vi "Dashboard Main.vi"() -> ()   [LabVIEW 2015]
uses:
  <vilib>/Utility/miscctls.llb/LVRowAndColumnTypeDef.ctl
  <vilib>/event_ctls.llb/eventvkey.ctl
  <vilib>/Rock Robotics/WPI/Dashboard/WPI_DashboardLogging Global.vi
  <vilib>/Rock Robotics/Network Tables/NT Read Numeric Array.vi
  <vilib>/Rock Robotics/Network Tables/NT Read Boolean.vi
  <vilib>/Utility/config.llb/Write Key (String).vi
  <vilib>/Utility/config.llb/Write Key (I32).vi
  <vilib>/Utility/config.llb/NI_LVConfig.lvlib
panel:
  in  "TCP":refnum<k5>
  in  "Rec Mode":enum32{"Stop", "Record", "Playback"}(radio)
  in  "Vision":u16(ring) items=["Camera Off", "USB Camera SW", "USB Camera HW", "IP Camera"]
  out "Camera IP":string
  out "Image Message":string="Timeout in Camera Communications"
  in  "Dashboard Tab":T1(tab)
  out "TANK":bool
  out "NT Connected":bool
  in  "Camera Settings":T2={"Frame Rate"=30, "Compression"=30, "Size"=1} {"Frame Rate" scale=1.0..30.0; "Size" items=["640x480", "320x240", "160x120"]}
  out "MotorChart R":cluster{"Numeric":dbl, "Numeric":dbl}(graph)
  out "MotorChart L":T3(graph)
  out "MotorSliders R":cluster{"MotorSlide1":dbl, "MotorSlide2":dbl} {"MotorSlide2" scale=-1.0..1.0 scale format="%#_2e"; "MotorSlide1" scale=-1.0..1.0 scale format="%#_2e"}
  out "MotorSliders L":T4 {"MotorSlide4 2" scale=0.0..14.0 scale format="%#_2e"; "MotorSlide2" scale=-1.0..1.0 scale format="%#_2e"; "MotorSlide1" scale=-1.0..1.0 scale format="%#_2e"}
  out "Gyro":dbl(knob) scale=0.0..360.0
  out "JS1 Z":dbl(slide) scale=-1.0..1.0 scale format="%#_2e"
  out "JS1 Graph":cluster{"X":dbl, "Y":dbl}[](graph)
  out "JS1 Buttons":T5
  out "JS2 Z":dbl(slide) scale=-1.0..1.0 scale format="%#_2e"
  out "JS2 Graph":cluster{"X":dbl, "Y":dbl}[](graph)
  out "JS2 Buttons":T5
  out "Mode":T6(ring)=enum."Auto Disabled"
  in  "DB Camera Config":bool
  out "fps":dbl format="%#.1g"
  out "Mbps":dbl format="%#.1g"
  out "Mbps 2":bool
  in  "DB/String 9":string
  in  "DB/String 8":string
  in  "DB/String 7":string
  in  "DB/String 6":string
  in  "DB/String 5":string
  in  "DB/String 4":string
  in  "DB/String 3":string
  in  "DB/String 2":string
  in  "DB/String 1":string
  in  "DB/String 0":string
  in  "DB/Slider 0":dbl(slide) scale=0.0..5.0
  in  "DB/Slider 1":dbl(slide) scale=0.0..5.0
  in  "DB/Slider 2":dbl(slide) scale=0.0..5.0
  in  "DB/Slider 3":dbl(slide) scale=0.0..5.0
  out "DB/LED 3":bool
  out "DB/LED 2":bool
  out "DB/LED 1":bool
  out "DB/LED 0":bool
  in  "DB/Button 3":bool
  in  "DB/Button 2":bool
  in  "DB/Button 1":bool
  in  "DB/Button 0":bool caption="New Name"
  in  "Test Slider":dbl(slide) scale=0.0..100.0 scale format="%#_3g"
  in  "On/Off":bool caption="Solenoid"
  in  "Test Name":u16(ring) items=["Select the test to run..."]
  in  "Test Tree":string(tree)
  in  "Motor":cluster{"Value":dbl, "Enable":bool} {"Value" scale=-1.0..1.0 scale format="%#_3g"}
  out "Progress":T7 {"Test Progress" scale=0.0..100.0}
  in  "Rev/Fwd":cluster{"Forward":bool, "Reverse":bool}
  in  "Test Ring":u16(ring) items=["Monochrome", "Color"]
  out "Cmd Status":string
  in  "Execute Command":bool
  in  "Command Params":string[][](table)
  in  "Command Selection":i32(listbox)
  in  "CheckList":i32(listbox)
  out "Tree":string(tree)
  out "Camera Image":T8(plugin-control)
  out "Boolean":bool
  # "Left"
  # "Front"
  # "Right"
  # "Battery"
  # "This tab is a great place for autonomous settings and robot-specific values.\nPlace controls and indicators inside this tab and match name to\nDashboard Variables on robot. You can also delete this comment."
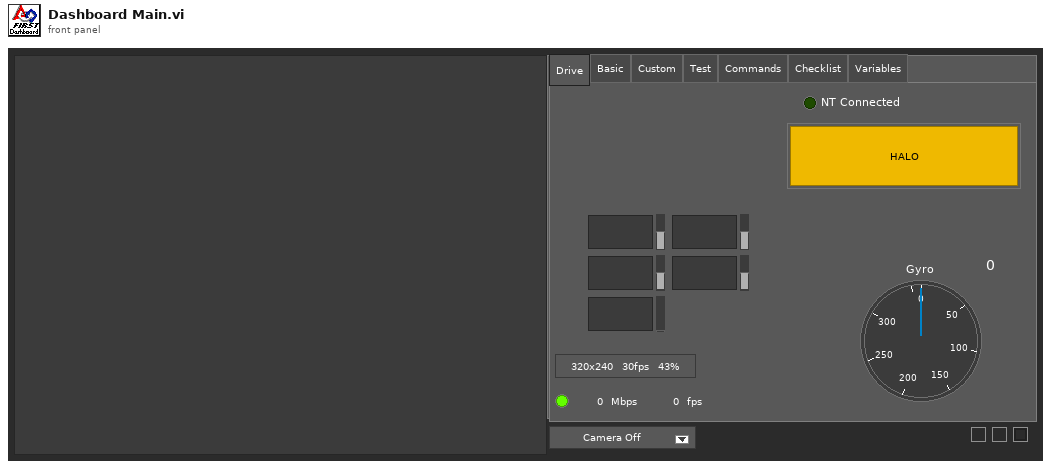
[diagram p1: front panel]
types:
  T1 = enum32{"Drive", "Basic", "Custom", "Test", "Commands", "Checklist", "Variables"}
  T2 = cluster{"Frame Rate":i32, "Compression":i32, "Size":u16}
  T3 = cluster{"Numeric":dbl, "Numeric":dbl, "Battery V":dbl}
  T4 = cluster{"MotorSlide1":dbl, "MotorSlide2":dbl, "MotorSlide4 2":dbl}
  T5 = cluster{bool, bool, bool, bool, bool, bool, bool, bool, bool, bool, bool, bool}
  T6 = enum8{"Tele-Op Disabled", "Tele-Op Enabled", "Auto Disabled", "Auto Enabled", "Test Disabled", "Test Enabled", "Disconnected", "No Code", "E-Stop"}
  T7 = cluster{"Test Progress":u8, "Test Progress Text":string}
  T8 = typedef "IMAQ Image.ctl" = refnum<image>
  T9 = cluster{"IDs":cluster{"RPC field ID":u16, "Unique ID":u16}, "String":string}
  T10 = enum32{"Drive", "Basic", "Custom", "Test", "Checklist", "Variables"}
  T11 = typedef "Image Type" = u32
  T12 = cluster{"Camera Image":refnum<vi>, "Dashboard Tab":refnum<vi>, "Boolean":refnum<vi>, "Vision":refnum<vi>, "Rec Mode":refnum<vi>, "Test Slider":refnum<vi>, "On/Off ":refnum<vi>, "Test Ring":refnum<vi>, "Rev/Fwd":refnum<vi>, "Test Name":refnum<vi>, "Motor":refnum<vi>, "Progress":refnum<vi>, "CheckList":refnum<vi>, "Tree":refnum<vi>, "Test Tree":refnum<vi>, "Command Params":refnum<vi>, "Command Selection":refnum<vi>, "Execute Command":refnum<vi>, "Cmd Status":refnum<vi>}
  T13 = cluster{"Error Strings":string, "Disable Counts":cluster{u16, u16}, "Rail Faults":cluster{u16, u16, u16}, "Robot IP":string, "DB Mode":u8, "Event Info":cluster{"Name":string, "Type":u8, "Number":u16, "Replay":u8}, "Camera Addr":string}
  T14 = cluster{"Storage":cluster{"Disk Free":u64, "RAM Block":u32, "RAM free":u32}, "CPU Utilization":cluster{"CPU % ISR":sgl, "CPU % Time Crit":sgl, "CPU % Timed Str":sgl, "CPU % High":sgl, "CPU % Above":sgl, "CPU % Normal":sgl, "CPU % Low":sgl}, "CAN":cluster{"% Bus Utilization":sgl, "Bus Off Cnt":u32, "TX_FIFO Full Cnt":u32, "Receive Error Cnt":u8, "Transmit Error Cnt":u8}, "HID":cluster{"HID Outputs":u32, "Rumble Low":u16, "Rumble High":u16}[]}
  T15 = cluster{"Status bits":cluster{"Test Mode":bool, "Autonomous":bool, "Enabled":bool, "Code Start":bool, "Brownout":bool, "Reserved 2":bool, "Reserved 3":bool, "E-Stop":bool}, "Code Trace":cluster{"Disabled":bool, "TeleOp":bool, "Auto":bool, "Test":bool}, "Controller Type":enum16{"unknown", "cRIO", "roboRio"}, "Code?":enum16{"unknown", "noCode", "code"}, "Battery V":dbl}
  T16 = cluster{"Control Bits":cluster{"TestMode":bool, "Autonomous":bool, "Enabled":bool, "FMS Present":bool, bool, bool, bool, "E-Stop":bool}, "Team Station ":u8, "Countdown":sgl, "Joystick Values":cluster{"Axes":dbl[], "Buttons":bool[], "POVs":i16[]}[]}
  T17 = cluster{"Axes":dbl[], "Buttons":bool[], "POVs":i16[]}[]
  T18 = cluster{"Axes":dbl[], "Buttons":bool[], "POVs":i16[]}
  T19 = cluster{"Buttons[0]":bool, "Buttons[1]":bool, "Buttons[2]":bool, "Buttons[3]":bool, "Buttons[4]":bool, "Buttons[5]":bool, "Buttons[6]":bool, "Buttons[7]":bool, "Buttons[8]":bool, "Buttons[9]":bool, "Buttons[10]":bool, "Buttons[11]":bool}
  T20 = typedef "NI_LVConfig.lvlib/Config Data RefNum.ctl" = refnum<k1>
  T21 = cluster{"Operation":enum16{"Update", "Clear"}, "Color Box":u32}[]
  T22 = typedef "eventvkey.ctl" = enum16{"ASCII", "Enter", "Return", "Shift", "Ctrl", "Alt", "Cmd", "Opt", "Caps", "NumLock", "Clear", "Break", "Up", "Down", "Left", "Right", "Insert", "Delete", "Home", "End", "PageUp", "PageDown", "Escape", "Help", "Pause", "ScrollLock", "F1", "F2", "F3", "F4", "F5", "F6", "F7", "F8", "F9", "F10", "F11", "F12", "F13", "F14", "F15", "F16", "F17", "F18", "F19", "F20", "F21", "F22", "F23", "F24", "Play", "VolumeUp", "VolumeDown", "Mute", "Two Byte Char"}
  T23 = cluster{"Image Size":bool, "Image Type":bool, "Pixel Value":bool, "ROI Information":bool, "Zoom Factor":bool}
  T24 = enum8{"Enabled", "Disabled", "Disabled and Grayed Out"}
  T25 = cluster{"Operation":enum16{"Update", "Clear"}, "Color Box":u32}
  T26 = typedef "LVRowAndColumnTypeDef.ctl" = cluster{"Row":i32, "Column":i32}
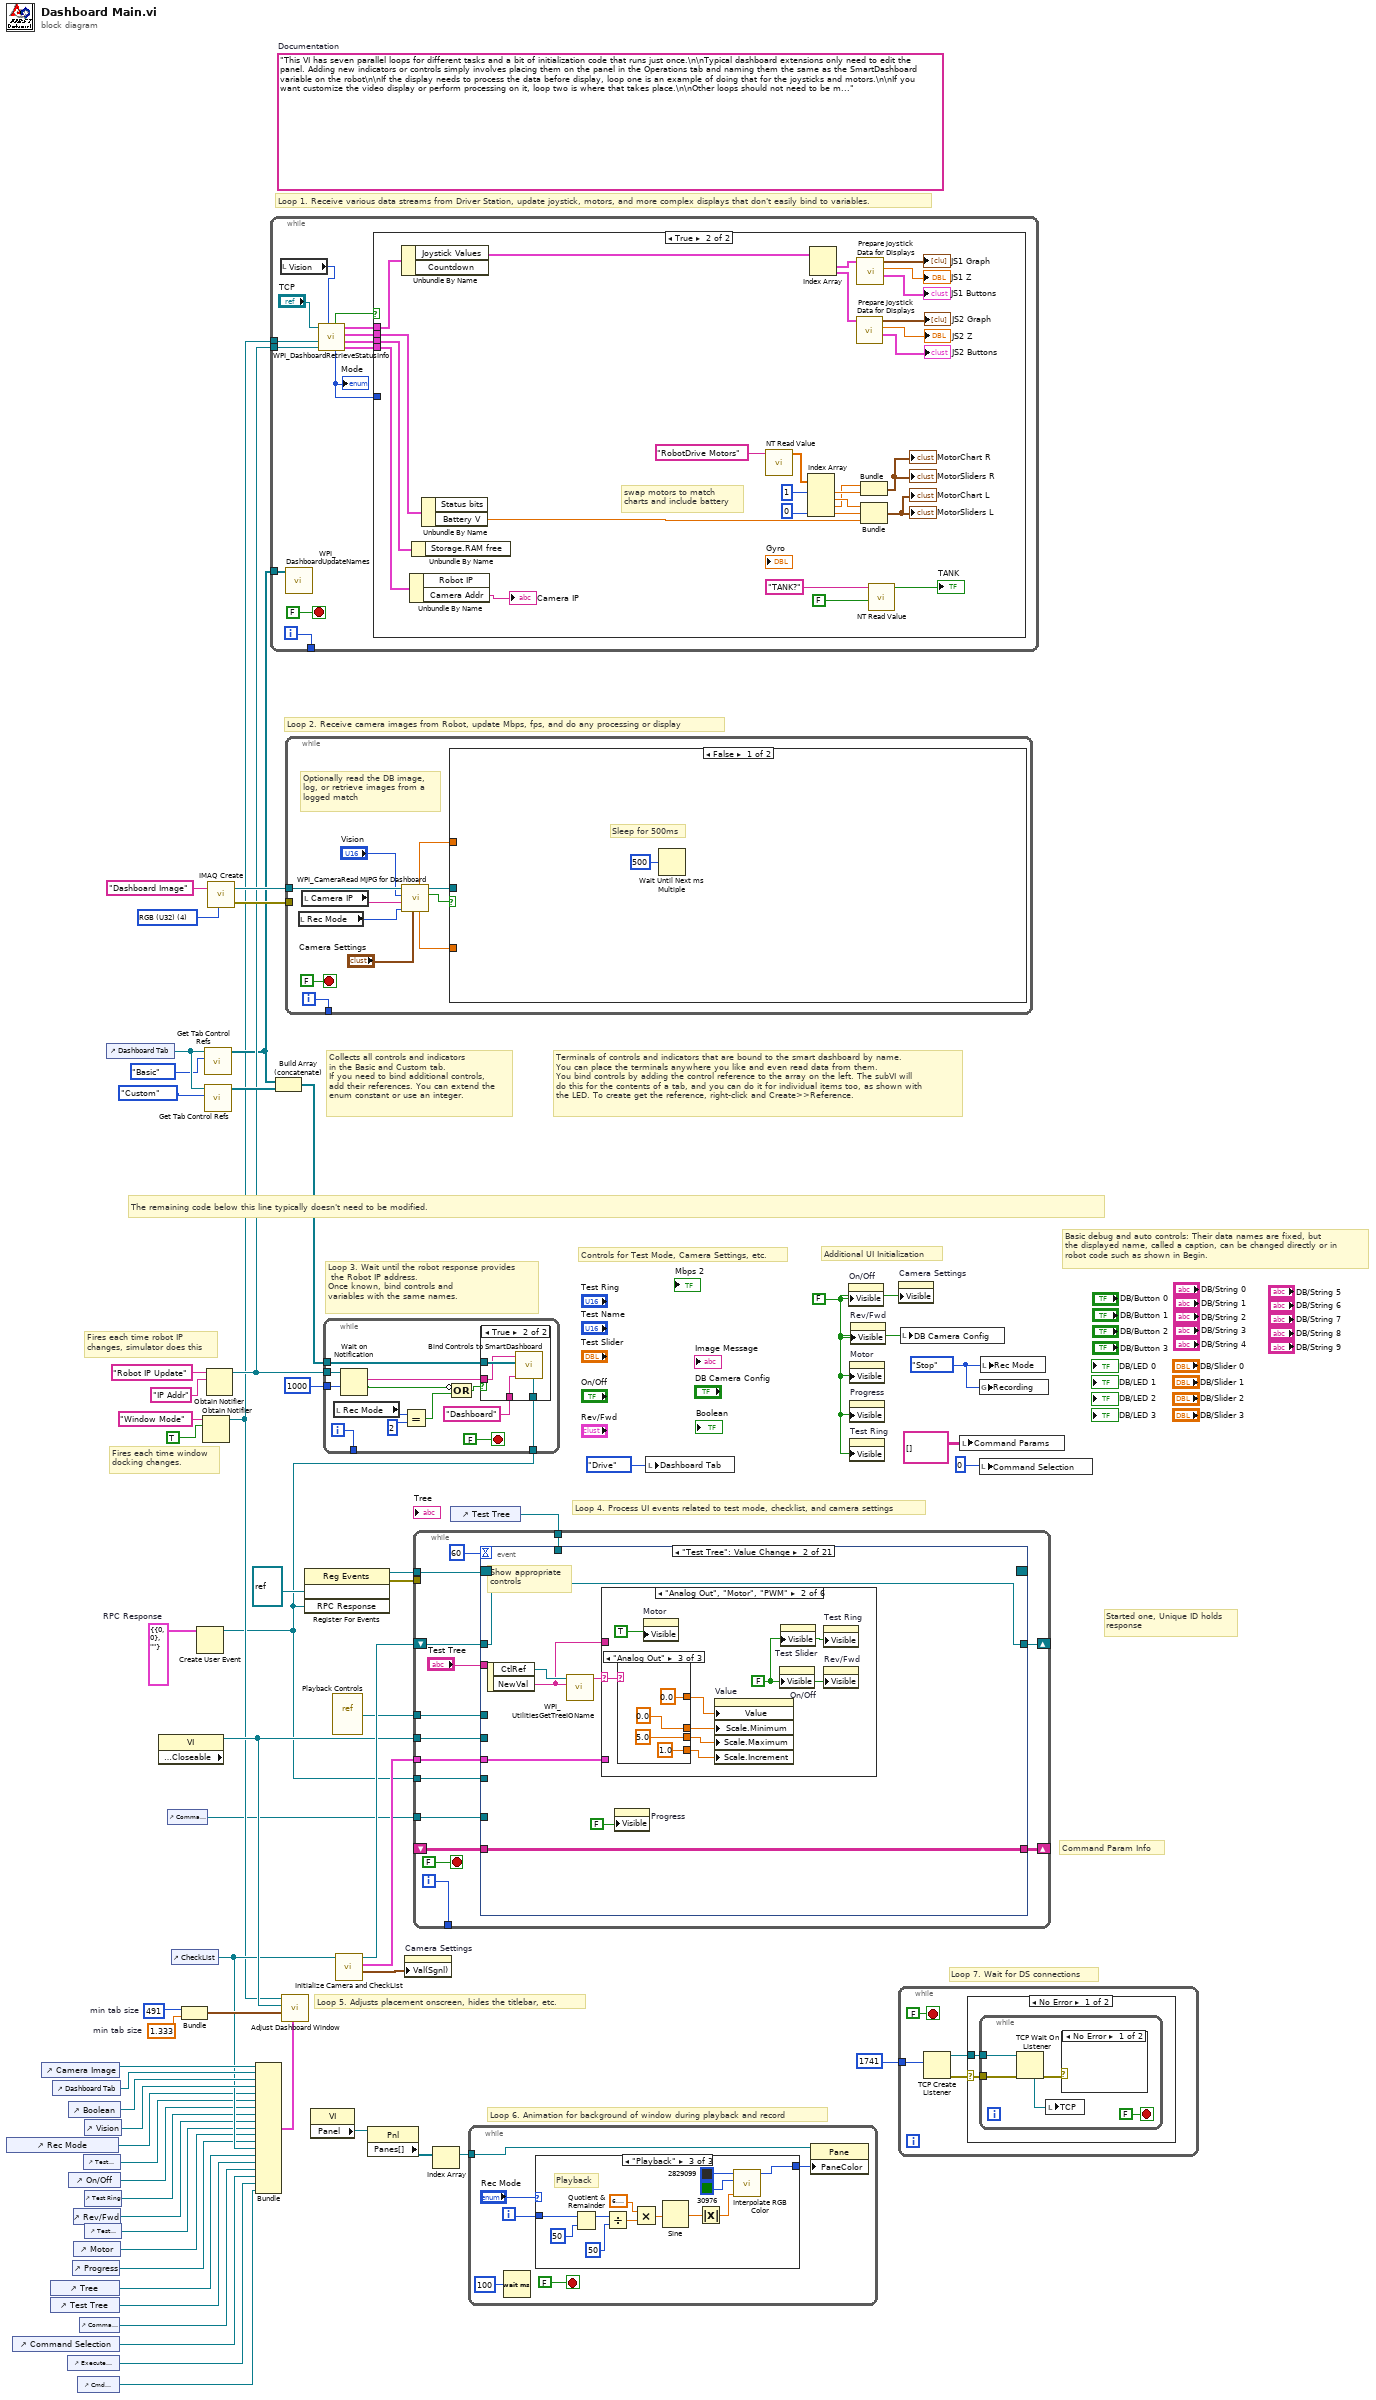
[diagram p0: block diagram]
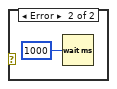
[diagram p2: hidden frame]
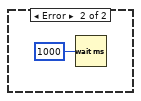
[diagram p3: hidden frame]
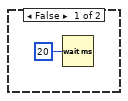
[diagram p4: hidden frame]
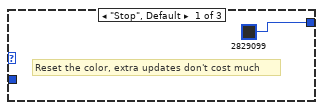
[diagram p5: hidden frame]
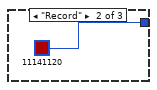
[diagram p6: hidden frame]
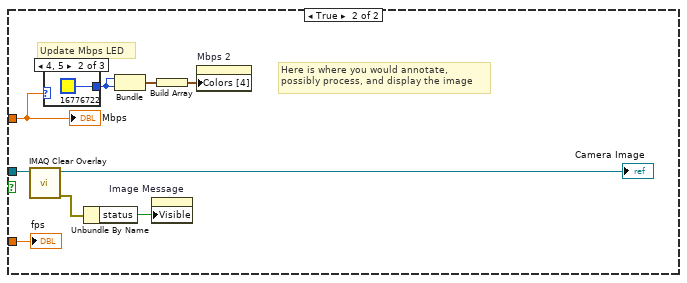
[diagram p8: hidden frame]
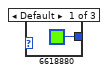
[diagram p9: hidden frame]
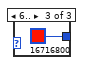
[diagram p10: hidden frame]
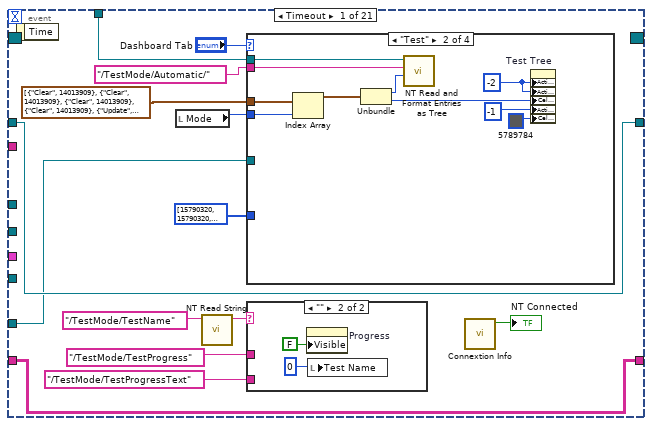
[diagram p11: hidden frame]
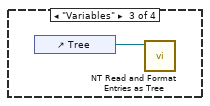
[diagram p13: hidden frame]
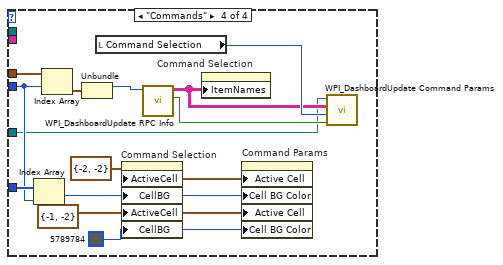
[diagram p14: hidden frame]
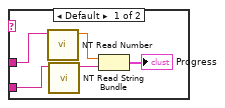
[diagram p15: hidden frame]
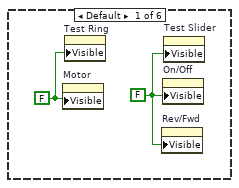
[diagram p16: hidden frame]
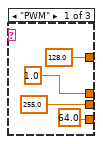
[diagram p17: hidden frame]
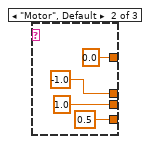
[diagram p18: hidden frame]
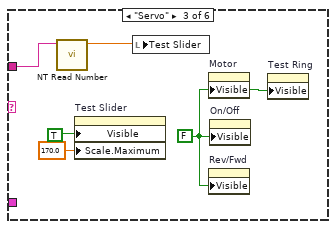
[diagram p19: hidden frame]
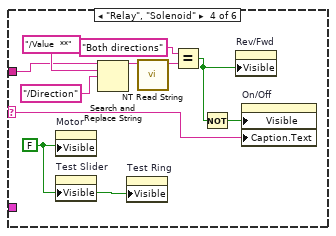
[diagram p20: hidden frame]
diagram:
  w7 = T9 {"IDs"={"RPC field ID"=0, "Unique ID"=0}, "String"=""}  # RPC Response
  w33 = 491  # min tab size
  w32 = 1.333  # min tab size
  w41 = enum32{"Stop", "Record", "Playback"}."Stop" ("Rec Mode")
  w15 = FALSE ("Visible")
  (unwired) "This VI has seven parallel loops for different tasks and a bit of initialization code that runs just once.\n\nTypical dashboard extensions only need to edit the panel. Adding new indicators or controls simply involves placing them on the panel in the Operations tab and naming them the same as the SmartDashboard variable on the robot\n\nIf the display needs to process the data before display, loop one is an example of doing that for the joysticks and motors.\n\nIf you want customize the video display or perform processing on it, loop two is where that takes place.\n\nOther loops should not need to be modified. They are pretty standard, and document the task they perform."  # Documentation
  w61 = T11 4 items=["Grayscale (U8)", "Grayscale (I16)", "Grayscale (SGL)", "Complex (CSG)", "RGB (U32)", "HSL (U32)", "RGB (U64)"] ("Image Type")
  # "Command Param Info"
  # "Started one, Unique ID holds\nresponse"
  # "Loop 7. Wait for DS connections"
  # "Basic debug and auto controls: Their data names are fixed, but\nthe displayed name, called a caption, can be changed directly or in\nrobot code such as shown in Begin."
  # "Controls for Test Mode, Camera Settings, etc."
  # "Additional UI Initialization"
  # "Loop 6. Animation for background of window during playback and record"
  # "Fires each time robot IP\nchanges, simulator does this"
  # "Fires each time window\ndocking changes."
  # "Collects all controls and indicators\nin the Basic and Custom tab.\nIf you need to bind additional controls,\nadd their references. You can extend the\nenum constant or use an integer."
  # "The remaining code below this line typically doesn't need to be modified."
  # "Loop 4. Process UI events related to test mode, checklist, and camera settings"
  # "Terminals of controls and indicators that are bound to the smart dashboard by name.\nYou can place the terminals anywhere you like and even read data from them.\nYou bind controls by adding the control reference to the array on the left. The subVI will\ndo this for the contents of a tab, and you can do it for individual items too, as shown with\nthe LED. To create get the reference, right-click and Create>>Reference."
  # "Loop 3. Wait until the robot response provides\n the Robot IP address.\nOnce known, bind controls and\nvariables with the same names."
  # "Loop 5. Adjusts placement onscreen, hides the titlebar, etc."
  # "Loop 1. Receive various data streams from Driver Station, update joystick, motors, and more complex displays that don't easily bind to variables."
  # "Loop 2. Receive camera images from Robot, update Mbps, fps, and do any processing or display"
  n1 = control-ref of="Rec Mode"() -> (w21:refnum<vi>)
  n2 = control-ref of="Command Selection"() -> (w6:refnum<vi>)
  n3 = control-ref of="Camera Image"() -> (w36:refnum<vi>)
  n4 = control-ref of="Tree"() -> (w25:refnum<vi>)
  n5 = control-ref of="Test Tree"() -> (w24:refnum<vi>)
  n6 = control-ref of="Dashboard Tab"() -> (w35:refnum<vi>)
  n7 = control-ref of="Execute Command"() -> (w8:refnum<vi>)
  n8 = control-ref of="Boolean"() -> (w30:refnum<vi>)
  n9 = control-ref of="On/Off"() -> (w19:refnum<vi>)
  n10 = control-ref of="Progress"() -> (w16:refnum<vi>)
  n11 = control-ref of="Rev/Fwd"() -> (w17:refnum<vi>)
  n12 = control-ref of="Motor"() -> (w22:refnum<vi>)
  n13 = control-ref of="Cmd Status"() -> (w2:refnum<vi>)
  n14 = control-ref of="Command Params"() -> (w9:refnum<vi>)
  n15 = control-ref of="Test Slider"() -> (w20:refnum<vi>)
  n16 = control-ref of="Vision"() -> (w34:refnum<vi>)
  n17 = control-ref of="Test Ring"() -> (w18:refnum<vi>)
  n18 = control-ref of="Test Name"() -> (w23:refnum<vi>)
  n19 = control-ref of="Dashboard Tab"() -> (w39:refnum<vi>)
  n20 = property class="VI" props=["Front Panel.Closeable"]() -> (reference out=w40:refnum<vi>)  [unwired: 2 in, 2 out]
  n21 = control-ref of="Command Params"() -> (w1:refnum<vi>)
  n22 = control-ref of="CheckList"() -> (w26:refnum<vi>)
  n23 = Bundle("min tab size"=w33, "min tab size"=w32) -> (w31:cluster{"min tab size":i32, "min tab size":dbl})  [unwired: 1 in]
  n24 = Create User Event(user event datatype=w7) -> (user event=w3:refnum<user-event>)  [unwired: 1 in, 1 out]
  n25 = Obtain Notifier(name (unnamed)="Window Mode", notification data type=TRUE) -> (notifier out=w12:refnum<notifier>)  [unwired: 2 in, 2 out]
  n26 = call <vilib>:"Get Tab Control Refs.vi"("Page Index"=T10."Basic" ("Dashboard Tab"), "TabControl in"=w39) -> ("ControlsOnPage"=w13:refnum<vi>[])  [unwired: 9 in]
  n27 = call <vilib>:"Get Tab Control Refs.vi"("Page Index"=T10."Custom" ("Dashboard Tab"), "TabControl in"=w39) -> ("ControlsOnPage"=w38:refnum<vi>[])  [unwired: 9 in]
  n28 = Obtain Notifier(name (unnamed)="Robot IP Update", notification data type="IP Addr" ("name (unnamed)")) -> (notifier out=w14:refnum<notifier>)  [unwired: 2 in, 2 out]
  n29 = call "IMAQ Create"("Image Name"="Dashboard Image", "Image Type"=w61) -> ("New Image"=w59:T8, "error out"=w58:errorcluster)  [unwired: 2 in, 1 out]
  n30 = Bundle("Camera Image"=w36, "Dashboard Tab"=w35, "Boolean"=w30, "Vision"=w34, "Rec Mode"=w21, "Test Slider"=w20, "On/Off"=w19, "Test Ring"=w18, "Rev/Fwd"=w17, "Test Name"=w23, "Motor"=w22, "Progress"=w16, "CheckList"=w26, "Tree"=w25, "Test Tree"=w24, "Command Params"=w9, "Command Selection"=w6, "Execute Command"=w8, "Cmd Status"=w2) -> (w27:T12)  [unwired: 1 in]
  n31 = while {
    tunnel: [w73] -> _
    tunnel: w14 -> [w67]
    tunnel: w13 -> [w66]
    tunnel: w12 -> [w62]
    i -> [w73]
    stop <- FALSE stop-if-true
    n32 = local read "Vision"() -> (w64:u16)
    n33 = call <vilib>:"WPI_DashboardUpdateNames.vi"("Controls on Tab"=w66) -> ()  [unwired: 11 in]
    n34 = call <vilib>:"WPI_DashboardRetrieveStatusInfo.vi"("Vision"=w64, "Binding Refnum"=w67, "Window Mode Notifier"=w62, "TCP Cnx"="TCP") -> ("Power and Errors"=w68:T13, "Robot Metrics"=w71:T14, "Status Info"=w72:T15, "Control Info"=w69:T16, "Robot Mode"=w65:T6, "Process?"=w70:bool)  [unwired: 2 in]
    "Mode" <- w65
    n35 = case shown="True" w70 {
      tunnel: w72 -> [_ w103]
      tunnel: w71 -> [_ w102]
      tunnel: w69 -> [_ w101]
      tunnel: w68 -> [_ w100]
      tunnel: w65 -> [_ _]
      frame False {
        n36 = Wait (ms)(milliseconds to wait=u32 20) -> ()  [unwired: 1 out]
      }
      frame True {
        # "swap motors to match\ncharts and include battery"
        n37 = Unbundle By Name(w101) -> ("Joystick Values"=w90:T17)  [unwired: 1 out]
        n38 = Unbundle By Name(w100) -> ("Camera Addr"=→"Camera IP":string)  [unwired: 1 out]
        n39 = Unbundle By Name(w102) -> ()  [unwired: 1 out]
        n40 = Unbundle By Name(w103) -> ("Battery V"=w91:dbl)  [unwired: 1 out]
        n41 = call-poly <vilib>:"NT Read Value.vi"("Name"="RobotDrive Motors") -> ("Numeric Array"=w79:dbl[])  [unwired: 9 in, 1 out]
        n42 = Index Array(array=w79, index #1=1, index #4=0) -> (element #1=w95:dbl, element #2=w96:dbl, element #3=w94:dbl, element #4=w99:dbl)  [unwired: 2 in]
        n43 = Index Array(array=w90) -> (element #1=w89:T18, element #2=w84:T18)  [unwired: 2 in]
        n44 = call "Prepare Joystick Data for Displays.vi"("Joystick Values"=w84) -> ("Buttons"=→"JS2 Buttons":T19, "Z Axis"=→"JS2 Z":dbl, "Cartesian Data"=→"JS2 Graph":cluster{"X axis":dbl, "X axis":dbl}[])  [unwired: 8 in]
        n45 = call "Prepare Joystick Data for Displays.vi"("Joystick Values"=w89) -> ("Buttons"=→"JS1 Buttons":T19, "Z Axis"=→"JS1 Z":dbl, "Cartesian Data"=→"JS1 Graph":cluster{"X axis":dbl, "X axis":dbl}[])  [unwired: 8 in]
        n46 = Bundle("Numeric"=w94, "Numeric"=w95) -> (→"MotorChart R" →"MotorSliders R":cluster{"Numeric":dbl, "Numeric":dbl})  [unwired: 1 in]
        n47 = Bundle("Numeric"=w96, "Numeric"=w99, "Battery V"=w91) -> (→"MotorChart L" →"MotorSliders L":T3)  [unwired: 1 in]
        n48 = call-poly <vilib>:"NT Read Value.vi"("Default Value"=FALSE, "Name"="TANK?") -> ("Boolean"=→"TANK":bool)  [unwired: 8 in, 1 out]
      }
    }
  }
  n49 = Build Array (concatenate)(w13, w38) -> (w37:refnum<vi>[])
  n50 = call "Adjust Dashboard Window.vi"("Sizing Refnums"=w27, "Size Constraints"=w31, "VI"=w40, "WIn Mode"=w12) -> ()  [unwired: 8 in]
  n51 = while {
    tunnel: w59 -> [w112]
    tunnel: w58 -> [_]
    tunnel: [w113] -> _
    i -> [w113]
    stop <- FALSE stop-if-true
    # "Optionally read the DB image,\nlog, or retrieve images from a\nlogged match"
    n52 = local read "Rec Mode"() -> (w106:enum32{"Stop", "Record", "Playback"})
    n53 = local read "Camera IP"() -> (w104:string)
    n54 = call <vilib>:"WPI_CameraRead MJPG for Dashboard.vi"("Camera Settings"="Camera Settings", "Rec Mode"=w106, "Camera IP"=w104, "Camera Mode"="Vision", "Refnum in"=w112) -> ("Active"=w110:bool, "Refnum out"=w111:T8, "FPS"=w109:dbl, "Bandwidth (Mbps)"=w108:dbl)  [unwired: 3 in]
    n55 = case shown="False" w110 {
      tunnel: w111 -> [_ w119]
      tunnel: w108 -> [_ w118]
      tunnel: w109 -> [_ w116]
      frame False {
        # "Sleep for 500ms"
        n56 = Wait Until Next ms Multiple(millisecond multiple=u32 500) -> ()  [unwired: 1 out]
      }
      frame True {
        # "Here is where you would annotate,\npossibly process, and display the image"
        # "Update Mbps LED"
        n57 = call "IMAQ Clear Overlay"("Image"=w119) -> ("error out"=w123:errorcluster, "Image Out"=→"Camera Image":T8)  [unwired: 2 in, 7 out]
        n58 = case shown="4, 5" w118 {
          tunnel: [u32 6618880 ("Color Box") u32 16776722 ("Color Box") u32 16716800 ("Color Box")] -> w120
          frame Default {
          }
          frame 4, 5 {
          }
          frame 6.. {
          }
        }
        n59 = Unbundle By Name(w123) -> ("status"=w124:bool)
        n60 = Bundle("Color Box"=w120, "Color Box"=w120) -> (w122:cluster{"Color Box":u32, "Color Box":u32})  [unwired: 1 out]
        n61 = property on="Image Message" class="Str"("Visible"=w124) -> ()  [unwired: 2 in, 2 out]
        n62 = Build Array(w122) -> (w121:cluster{"Color Box":u32, "Color Box":u32}[])
        n63 = property on="Mbps 2" class="Bool (strict)"("Colors [4]"=w121) -> ()  [unwired: 2 in, 2 out]
        "Mbps" <- w118
        "fps" <- w116
      }
    }
  }
  n64 = register-events(refnum<vi> refnum, w3) -> (reference out=w45:refnum<event-registration>, error out=w44:errorcluster)  [unwired: 2 in]
  n65 = property class="VI"() -> ("Panel"=w48:refnum<vi>)  [unwired: 2 in, 2 out]
  n66 = while {
    tunnel: w37 -> [w140]
    tunnel: w14 -> [w138]
    tunnel: [w136] -> _
    tunnel: u32 1000 ("milliseconds to wait") -> [w135]
    tunnel: w3 -> [w128]
    i -> [w136]
    stop <- FALSE stop-if-true
    n67 = local read "Rec Mode"() -> (w131:enum32{"Stop", "Record", "Playback"})
    n68 = Wait on Notification(notifier=w138, timeout in ms (-1)=w135) -> (notification=w137:string, timed out?=w133:bool)  [unwired: 2 in, 2 out]
    n69 = Equal?(x=w131, y=u16 2 ("Rec Mode")) -> (x = y?=w132:bool)
    n70 = Compound Arithmetic op=OR(invert w133, w132) -> (w134:bool)
    n71 = case shown="True" w134 {
      tunnel: w140 -> [_ w144]
      tunnel: w137 -> [_ w143]
      tunnel: "Dashboard" -> [_ w142]
      tunnel: w128 -> [_ w141]
      frame False {
      }
      frame True {
        n72 = call <vilib>:"Bind Controls to SmartDashboard.vi"("RPC ref"=w141, "Client Name"=w142, "Bound Control Refs"=w144, "Server IP Address"=w143) -> ()  [unwired: 8 in]
      }
    }
  }
  n73 = vi-ref "Playback Controls.vi"() -> (w46:refnum<vi>)
  n74 = call "Initialize Camera and CheckList.vi"("ListBox in"=w26) -> ("Cluster"=w52:cluster{"value":i32, "value":i32, "index":i32}, "Array"=w53:cluster{string[]}[], "File Refnum"=w51:T20)  [unwired: 8 in]
  n75 = property class="Pnl"(reference=w48) -> ("Panes[]"=w49:refnum<vi>[])  [unwired: 1 in, 2 out]
  n76 = property on="Camera Settings" class="Clust (strict)"("Val(Sgnl)"=w52) -> ()  [unwired: 2 in, 2 out]
  n77 = Index Array(array=w49) -> (element=w47:refnum<vi>)  [unwired: 1 in]
  n78 = control-ref of="Test Tree"() -> (w50:refnum<vi>)
  n79 = while {
    tunnel: w53 -> [w156]
    shift-right: [w155] -> _
    shift-left: w51 -> [w154]
    tunnel: [w153] -> _
    tunnel: w50 -> [w152]
    tunnel: w46 -> [w151]
    tunnel: w45 -> [w150]
    tunnel: w44 -> [_]
    tunnel: w40 -> [w149]
    tunnel: w3 -> [w148]
    tunnel: w1 -> [w147]
    shift-right: [w146] -> _
    shift-left: _ -> [w145]
    i -> [w153]
    stop <- FALSE stop-if-true
    n80 = event shown="[1] \"Test Tree\": Value Change" {
      selector: w150 -> [_ _ _ _ _ _ _ _ _ _ _ _ _ _ _ _ _ _ _ _ _]
      dyn-events: [_ _ _ _ _ _ _ _ _ _ _ _ _ _ _ _ w457 _ _ _ _] -> _
      timeout: u32 60 ("milliseconds to wait") -> [_ _ _ _ _ _ _ _ _ _ _ _ _ _ _ _ _ _ _ _ _]
      tunnel: w152 -> [w169 _ _ _ _ _ _ _ _ _ _ _ _ _ _ _ _ _ _ _ _]
      tunnel: "Test Tree" -> [_ _ _ _ _ _ _ _ _ _ _ w420 w429 w432 w437 w446 _ _ _ _ _]
      tunnel: w156 -> [_ w207 _ _ _ _ _ _ _ w382 w413 _ _ _ _ _ _ _ _ _ _]
      tunnel: [w166 w206 w310 w316 w328 w340 w348 w354 w367 w381 w406 w419 w427 w431 w436 w445 w459 w475 w477 w485 w496] -> w155
      tunnel: w154 -> [w166 w206 w310 w316 w328 w340 w348 w354 w367 w380 w406 w419 w427 w431 w436 w445 w459 w475 w477 w485 w496]
      tunnel: w151 -> [_ _ _ _ _ _ _ _ _ _ _ _ _ _ _ _ w460 _ w480 _ _]
      tunnel: w149 -> [_ _ _ _ _ _ _ _ _ _ _ _ _ _ _ _ w455 _ _ _ _]
      tunnel: w148 -> [_ _ _ _ _ _ _ _ _ _ _ _ _ _ _ _ w451 _ _ _ _]
      tunnel: w147 -> [w161 _ _ _ w326 _ _ _ _ _ _ _ _ _ _ _ _ _ _ _ _]
      tunnel: [w160 w205 w309 w315 w324 w334 w345 w353 w366 w379 w405 w418 w426 w430 w435 w444 w450 w473 w476 w481 w489] -> w146
      tunnel: w145 -> [w160 w205 w309 w315 w324 _ _ w353 w366 w379 w405 w418 w426 w430 w435 w444 w450 w473 w476 w481 w489]
      event Timeout {
        n81 = event-data() -> ()  [unwired: 1 in, 1 out]
        n82 = local read "Mode"() -> (w163:T6)
        n83 = call <vilib>:"NT Read String.vi"("Name"="/TestMode/TestName") -> ("String"=w172:string)  [unwired: 9 in, 1 out]
        n84 = case shown="\"Test\"" "Dashboard Tab" {
          tunnel: w169 -> [_ w183 _ _]
          tunnel: "/TestMode/Automatic/" ("Name Pattern") -> [_ w182 _ _]
          tunnel: T21 [{"Operation"=enum."Clear", "Color Box"=14013909}, {"Operation"=enum."Clear", "Color Box"=14013909}, {"Operation"=enum."Clear", "Color Box"=14013909}, {"Operation"=enum."Clear", "Color Box"=14013909}, {"Operation"=enum."Update", "Color Box"=14013909}, {"Operation"=enum."Update", "Color Box"=16777215}, {"Operation"=enum."Clear", "Color Box"=14013909}, {"Operation"=enum."Clear", "Color Box"=14013909}, {"Operation"=enum."Clear", "Color Box"=14013909}] -> [_ w175 _ w192]
          tunnel: w163 -> [_ w174 _ w191]
          tunnel: u32[] [15790320, 15790320, 15790320, 15790320, 16777215, 16777215, 15790320, 15790320, 15790320] -> [_ _ _ w197]
          tunnel: w161 -> [_ _ _ w185]
          frame "Custom", Default {
          }
          frame "Test" {
            w181 = -2 ("Active Item:Row Number")
            n85 = Index Array(array=w175, index=w174) -> (element=w176:T25)
            n86 = Unbundle(w176) -> ("Operation"=w177:enum16{"Update", "Clear"}, "Color Box"=w178:u32)
            n87 = call <vilib>:"NT Read and Format Entries as Tree.vi"("Operation"=w177, "Name Pattern"=w182, "Tree Refnum"=w183) -> ()  [unwired: 7 in, 2 out]
            n88 = property on="Test Tree" class="Tree (strict)"("Active Item Row Number"=w181, "ActiveColNum"=w181, "CellBG"=w178, "Active Item Row Number"=-1 ("Active Item:Row Number"), "CellBG"=u32 5789784 ("Color Box")) -> ()  [unwired: 2 in, 2 out]
          }
          frame "Variables" {
            n89 = control-ref of="Tree"() -> (w184:refnum<vi>)
            n90 = call <vilib>:"NT Read and Format Entries as Tree.vi"("Tree Refnum"=w184) -> ()  [unwired: 9 in, 2 out]
          }
          frame "Commands" {
            w193 = u32 5789784 ("Color Box")
            w194 = T26 {"Row"=-1, "Column"=-2} ("Active Cell:Active Cell")
            w196 = T26 {"Row"=-2, "Column"=-2} ("Active Cell:Active Cell")
            n91 = Index Array(array=w197, index=w191) -> (element=w195:u32)
            n92 = Index Array(array=w192, index=w191) -> (element=w190:T25)
            n93 = Unbundle(w190) -> ("Operation"=w189:enum16{"Update", "Clear"})  [unwired: 1 out]
            n94 = local read "Command Selection"() -> (w188:i32)
            n95 = property on="Command Selection" class="MCListbox (strict)"("ActiveCell"=w196, "CellBG"=w195, "ActiveCell"=w194, "CellBG"=w193) -> ()  [unwired: 2 in, 2 out]
            n96 = call <vilib>:"WPI_DashboardUpdate RPC Info.vi"("Operation"=w189) -> ("update"=w187:bool, "commands"=w186:string[][])  [unwired: 9 in]
            n97 = property on="Command Selection" class="MCListbox (strict)"("ItemNames"=w186) -> ()  [unwired: 2 in, 2 out]
            n98 = property on="Command Params" class="Tbl (strict)"("Active Cell"=w196, "Cell BG Color"=w195, "Active Cell"=w194, "Cell BG Color"=w193) -> ()  [unwired: 2 in, 2 out]
            n99 = call <vilib>:"WPI_DashboardUpdate Command Params.vi"("Update"=w187, "NewVal"=w188, "Commands"=w186, "Param Tbl"=w185) -> ()  [unwired: 7 in, 1 out]
          }
        }
        n100 = case shown="\"\"" w172 {
          tunnel: "/TestMode/TestProgress" ("Name") -> [w199 _]
          tunnel: "/TestMode/TestProgressText" ("Name") -> [w198 _]
          frame Default {
            n101 = call <vilib>:"NT Read Number.vi"("Name"=w199) -> ("Numeric"=w200:dbl)  [unwired: 9 in, 1 out]
            n102 = call <vilib>:"NT Read String.vi"("Name"=w198) -> ("String"=w201:string)  [unwired: 9 in, 1 out]
            n103 = Bundle("Numeric"=w200, "String"=w201) -> (→"Progress":cluster{"Numeric":dbl, "String":string})  [unwired: 1 in]
          }
          frame "" {
            n104 = property on="Progress" class="Clust (strict)"("Visible"=FALSE) -> ()  [unwired: 2 in, 2 out]
            n105 = local write "Test Name"(u16 0) -> ()
          }
        }
        n106 = call <vilib>:"Connextion Info.vi"() -> ("Connected"=→"NT Connected":bool)  [unwired: 10 in, 1 out]
      }
      event "Test Tree": Value Change {
        # "Show appropriate\ncontrols"
        n107 = event-data() -> ("CtlRef"=w210:refnum<vi>, "NewVal"=w208:string)  [unwired: 1 in]
        n108 = call <vilib>:"WPI_UtilitiesGetTreeIOName.vi"("NewVal"=w208, "TreeControl in"=w210) -> ("I/O Name"=w211:string)  [unwired: 9 in]
        n109 = case shown="\"Analog Out\", \"Motor\", \"PWM\"" w211 {
          selector: w211 -> [_ w218 _ w240 w249 _]
          tunnel: w208 -> [_ _ w237 w239 _ w256]
          tunnel: w207 -> [_ _ _ _ _ w255]
          frame Default {
            w213 = FALSE ("Visible")
            w212 = FALSE ("Visible")
            n110 = property on="Motor" class="Clust (strict)"("Visible"=w212) -> ()  [unwired: 2 in, 2 out]
            n111 = property on="Test Ring" class="Ring (strict)"("Visible"=w212) -> ()  [unwired: 2 in, 2 out]
            n112 = property on="Rev/Fwd" class="Clust (strict)"("Visible"=w213) -> ()  [unwired: 2 in, 2 out]
            n113 = property on="On/Off" class="Bool (strict)"("Visible"=w213) -> ()  [unwired: 2 in, 2 out]
            n114 = property on="Test Slider" class="Slide (strict)"("Visible"=w213) -> ()  [unwired: 2 in, 2 out]
          }
          frame "Analog Out", "Motor", "PWM" {
            w219 = FALSE ("Visible")
            n115 = case shown="\"Analog Out\"" w218 {
              tunnel: [1.0 ("Value") -1.0 ("Value") 0.0 ("Value")] -> w217
              tunnel: [255.0 ("Value") 1.0 ("Value") 5.0 ("Value")] -> w216
              tunnel: [128.0 ("Value") 0.0 ("Value") 0.0 ("Value")] -> w215
              tunnel: [64.0 ("Value") 0.5 ("Value") 1.0 ("Value")] -> w214
              frame "PWM" {
              }
              frame "Motor", Default {
              }
              frame "Analog Out" {
              }
            }
            n116 = property on="Motor" class="Clust (strict)"("Visible"=TRUE) -> ()  [unwired: 2 in, 2 out]
            n117 = property on="Value" class="Slide (strict)"("Value"=w215, "Scale.Minimum"=w217, "Scale.Maximum"=w216, "Scale.Increment"=w214) -> ()  [unwired: 2 in, 2 out]
            n118 = property on="On/Off" class="Bool (strict)"("Visible"=w219) -> ()  [unwired: 2 in, 2 out]
            n119 = property on="Test Slider" class="Slide (strict)"("Visible"=w219) -> ()  [unwired: 2 in, 2 out]
            n120 = property on="Test Ring" class="Ring (strict)"("Visible"=w219) -> ()  [unwired: 2 in, 2 out]
            n121 = property on="Rev/Fwd" class="Clust (strict)"("Visible"=w219) -> ()  [unwired: 2 in, 2 out]
          }
          frame "Servo" {
            w235 = FALSE ("Visible")
            n122 = call <vilib>:"NT Read Number.vi"("Name"=w237) -> ("Numeric"=w236:dbl)  [unwired: 9 in, 1 out]
            n123 = property on="Test Slider" class="Slide (strict)"("Visible"=TRUE, "Scale.Maximum"=170.0 ("Scale.Range:Maximum")) -> ()  [unwired: 2 in, 2 out]
            n124 = local write "Test Slider"(w236) -> ()
            n125 = property on="Motor" class="Clust (strict)"("Visible"=w235) -> ()  [unwired: 2 in, 2 out]
            n126 = property on="Rev/Fwd" class="Clust (strict)"("Visible"=w235) -> ()  [unwired: 2 in, 2 out]
            n127 = property on="On/Off" class="Bool (strict)"("Visible"=w235) -> ()  [unwired: 2 in, 2 out]
            n128 = property on="Test Ring" class="Ring (strict)"("Visible"=w235) -> ()  [unwired: 2 in, 2 out]
          }
          frame "Relay", "Solenoid" {
            w238 = FALSE ("Visible")
            n129 = property on="Motor" class="Clust (strict)"("Visible"=w238) -> ()  [unwired: 2 in, 2 out]
            n130 = property on="Test Slider" class="Slide (strict)"("Visible"=w238) -> ()  [unwired: 2 in, 2 out]
            n131 = Search and Replace String(input string=w239, search string="/Value  **", replace string="/Direction") -> (result string=w245:string)  [unwired: 5 in, 3 out]
            n132 = property on="Test Ring" class="Ring (strict)"("Visible"=w238) -> ()  [unwired: 2 in, 2 out]
            n133 = call <vilib>:"NT Read String.vi"("Name"=w245) -> ("String"=w243:string)  [unwired: 9 in, 1 out]
            n134 = Equal?(x="Both directions", y=w243) -> (x = y?=w241:bool)
            n135 = Not(x=w241) -> (.not. x?=w242:bool)
            n136 = property on="Rev/Fwd" class="Clust (strict)"("Visible"=w241) -> ()  [unwired: 2 in, 2 out]
            n137 = property on="On/Off" class="Bool (strict)"("Visible"=w242, "Caption.Text"=w240) -> ()  [unwired: 2 in, 2 out]
          }
          frame "Compressor", "Digital Out" {
            w248 = FALSE ("Visible")
            # "Get direction and finish"
            n138 = property on="Motor" class="Clust (strict)"("Visible"=w248) -> ()  [unwired: 2 in, 2 out]
            n139 = property on="Test Slider" class="Slide (strict)"("Visible"=w248) -> ()  [unwired: 2 in, 2 out]
            n140 = property on="Test Ring" class="Ring (strict)"("Visible"=w248) -> ()  [unwired: 2 in, 2 out]
            n141 = property on="On/Off" class="Bool (strict)"("Visible"=TRUE, "Caption.Text"=w249) -> ()  [unwired: 2 in, 2 out]
            n142 = property on="Rev/Fwd" class="Clust (strict)"("Visible"=FALSE) -> ()  [unwired: 2 in, 2 out]
          }
          frame "Camera" {
            n143 = call <vilib>:"Get Last Path Segment.vi"("String in"=w256) -> ("String out"=w257:string)  [unwired: 10 in]
            n144 = property on="On/Off" class="Bool (strict)"("Visible"=FALSE) -> ()  [unwired: 2 in, 2 out]
            n145 = property on="Motor" class="Clust (strict)"("Visible"=FALSE) -> ()  [unwired: 2 in, 2 out]
            n146 = property on="Rev/Fwd" class="Clust (strict)"("Visible"=FALSE) -> ()  [unwired: 2 in, 2 out]
            n147 = case shown="\"White Balance  **\"" w257 {
              tunnel: w256 -> [w263 w272 w281 w290 w299 _ w305]
              tunnel: w255 -> [w261 w269 w278 w287 w296 _ _]
              frame "Size  **" {
                n148 = Index Array(array=w261) -> (element=w260:cluster{string[]})  [unwired: 1 in]
                n149 = call <vilib>:"NT Read String.vi"("Name"=w263) -> ("String"=w262:string)  [unwired: 9 in, 1 out]
                n150 = Unbundle(w260) -> (w258:string[])
                n151 = Match First String(2:w258, 3:w262) -> (0:w259:i32)  [unwired: 1 out]
                n152 = property on="Test Ring" class="Ring (strict)"("Value"=w259, "Strings []"=w258) -> ()  [unwired: 2 in, 2 out]
                n153 = property on="Test Ring" class="Ring (strict)"("Visible"=TRUE) -> ()  [unwired: 2 in, 2 out]
                n154 = property on="Test Slider" class="Slide (strict)"("Visible"=FALSE) -> ()  [unwired: 2 in, 2 out]
              }
              frame "White Balance  **" {
                n155 = Index Array(array=w269, index=1) -> (element=w270:cluster{string[]})
                n156 = call <vilib>:"NT Read String.vi"("Name"=w272) -> ("String"=w271:string)  [unwired: 9 in, 1 out]
                n157 = Unbundle(w270) -> (w267:string[])
                n158 = Match First String(2:w267, 3:w271) -> (0:w266:i32)  [unwired: 1 out]
                n159 = property on="Test Ring" class="Ring (strict)"("Value"=w266, "Strings []"=w267) -> ()  [unwired: 2 in, 2 out]
                n160 = property on="Test Ring" class="Ring (strict)"("Visible"=TRUE) -> ()  [unwired: 2 in, 2 out]
                n161 = property on="Test Slider" class="Slide (strict)"("Visible"=FALSE) -> ()  [unwired: 2 in, 2 out]
              }
              frame "Exposure  **" {
                n162 = Index Array(array=w278, index=2) -> (element=w279:cluster{string[]})
                n163 = call <vilib>:"NT Read String.vi"("Name"=w281) -> ("String"=w280:string)  [unwired: 9 in, 1 out]
                n164 = Unbundle(w279) -> (w275:string[])
                n165 = Match First String(2:w275, 3:w280) -> (0:w276:i32)  [unwired: 1 out]
                n166 = property on="Test Ring" class="Ring (strict)"("Value"=w276, "Strings []"=w275) -> ()  [unwired: 2 in, 2 out]
                n167 = property on="Test Ring" class="Ring (strict)"("Visible"=TRUE) -> ()  [unwired: 2 in, 2 out]
                n168 = property on="Test Slider" class="Slide (strict)"("Visible"=FALSE) -> ()  [unwired: 2 in, 2 out]
              }
              frame "Exposure Priority  **" {
                n169 = Index Array(array=w287, index=3) -> (element=w288:cluster{string[]})
                n170 = call <vilib>:"NT Read String.vi"("Name"=w290) -> ("String"=w289:string)  [unwired: 9 in, 1 out]
                n171 = Unbundle(w288) -> (w284:string[])
                n172 = Match First String(2:w284, 3:w289) -> (0:w285:i32)  [unwired: 1 out]
                n173 = property on="Test Ring" class="Ring (strict)"("Value"=w285, "Strings []"=w284) -> ()  [unwired: 2 in, 2 out]
                n174 = property on="Test Ring" class="Ring (strict)"("Visible"=TRUE) -> ()  [unwired: 2 in, 2 out]
                n175 = property on="Test Slider" class="Slide (strict)"("Visible"=FALSE) -> ()  [unwired: 2 in, 2 out]
              }
              frame "Color Enable  **" {
                n176 = Index Array(array=w296, index=4) -> (element=w297:cluster{string[]})
                n177 = call <vilib>:"NT Read String.vi"("Name"=w299) -> ("String"=w298:string)  [unwired: 9 in, 1 out]
                n178 = Unbundle(w297) -> (w293:string[])
                n179 = Match First String(2:w293, 3:w298) -> (0:w294:i32)  [unwired: 1 out]
                n180 = property on="Test Ring" class="Ring (strict)"("Value"=w294, "Strings []"=w293) -> ()  [unwired: 2 in, 2 out]
                n181 = property on="Test Ring" class="Ring (strict)"("Visible"=TRUE) -> ()  [unwired: 2 in, 2 out]
                n182 = property on="Test Slider" class="Slide (strict)"("Visible"=FALSE) -> ()  [unwired: 2 in, 2 out]
              }
              frame Default {
                n183 = property on="Test Ring" class="Ring (strict)"("Visible"=FALSE) -> ()  [unwired: 2 in, 2 out]
                n184 = property on="Test Slider" class="Slide (strict)"("Visible"=FALSE) -> ()  [unwired: 2 in, 2 out]
              }
              frame "Brightness  **", "Color Level  **", "Compression  **", "FPS  **", "Sharpness  **" {
                n185 = call <vilib>:"NT Read Number.vi"("Name"=w305) -> ("Numeric"=w304:dbl)  [unwired: 9 in, 1 out]
                n186 = local write "Test Slider"(w304) -> ()
                n187 = property on="Test Slider" class="Slide (strict)"("Visible"=TRUE, "Scale.Maximum"=100.0 ("Scale.Range:Maximum")) -> ()  [unwired: 2 in, 2 out]
                n188 = property on="Test Ring" class="Ring (strict)"("Visible"=FALSE) -> ()  [unwired: 2 in, 2 out]
              }
            }
          }
        }
        n189 = property on="Progress" class="Clust (strict)"("Visible"=FALSE) -> ()  [unwired: 2 in, 2 out]
      }
      event "Test Name": Mouse Enter {
        # "Populate the ring with the list of tests"
        n190 = event-data() -> ()  [unwired: 1 in, 1 out]
        n191 = call <vilib>:"NT Read String Array.vi"("Name"="/TestMode/TestList") -> ("String Array"=w314:string[])  [unwired: 9 in, 1 out]
        n192 = Build Array (concatenate)("Select the test to run...", w314) -> (w313:string[])
        n193 = property on="Test Name" class="Ring (strict)"("Strings []"=w313) -> ()  [unwired: 2 in, 2 out]
      }
      event "Test Name": Value Change {
        w317 = FALSE ("Visible")
        # "Tell the robot the test name to run"
        n194 = event-data() -> ("NewVal"=w321:u16)  [unwired: 1 in]
        n195 = property on="Test Name" class="Ring (strict)"() -> ("Strings []"=w322:string[])  [unwired: 2 in, 2 out]
        n196 = local write "Progress"(T7 {"Test Progress"=0, "Test Progress Text"=""} ("Progress")) -> ()
        n197 = Index Array(array=w322, index=w321) -> (element=w320:string)
        n198 = call <vilib>:"NT Write String.vi"("String"=w320, "Name"="/TestMode/TestName") -> ()  [unwired: 9 in, 1 out]
        n199 = property on="Progress" class="Clust (strict)"("Visible"=TRUE) -> ()  [unwired: 2 in, 2 out]
        n200 = property on="Motor" class="Clust (strict)"("Visible"=w317) -> ()  [unwired: 2 in, 2 out]
        n201 = property on="Test Slider" class="Slide (strict)"("Visible"=w317) -> ()  [unwired: 2 in, 2 out]
        n202 = property on="On/Off" class="Bool (strict)"("Visible"=w317) -> ()  [unwired: 2 in, 2 out]
        n203 = property on="Rev/Fwd" class="Clust (strict)"("Visible"=w317) -> ()  [unwired: 2 in, 2 out]
        n204 = property on="Test Ring" class="Ring (strict)"("Visible"=w317) -> ()  [unwired: 2 in, 2 out]
      }
      event "Command Selection": Value Change {
        # "Get the params and show in table"
        n205 = event-data() -> ("NewVal"=w327:i32)  [unwired: 1 in]
        n206 = property on="Command Selection" class="MCListbox (strict)"() -> ("ItemNames"=w325:string[][])  [unwired: 2 in, 2 out]
        n207 = call <vilib>:"WPI_DashboardUpdate Command Params.vi"("NewVal"=w327, "Commands"=w325, "Param Tbl"=w326) -> ()  [unwired: 8 in, 1 out]
      }
      event "Execute Command": Value Change {
        # "Started one, Unique ID holds\nresponse"
        n208 = event-data() -> ()  [unwired: 1 in, 1 out]
        n209 = property on="Command Selection" class="MCListbox (strict)"() -> ("ItemNames"=w339:string[][])  [unwired: 2 in, 2 out]
        n210 = Index Array(array=w339, index (row)="Command Selection", index (col)=0) -> (element=w337:string)
        n211 = call <vilib>:"Invoke Commands.vi"("Command Params"="Command Params", "Function Name"=w337) -> ("Params"=w333:u8, "Started"=w332:bool)  [unwired: 7 in, 1 out]
        n212 = Array Subset(array="Command Params", length (row)=w333) -> (w334:string[][])  [unwired: 3 in]
        n213 = Select(t="Executing" ("Cmd Status"), s=w332, f="" ("Cmd Status")) -> (s? t:f=→"Cmd Status":string)
      }
      event "Command Selection": Double Click {
        n214 = event-data() -> ("Row"=w349:i32)  [unwired: 1 in]
        n215 = property on="Command Selection" class="MCListbox (strict)"() -> ("ItemNames"=w352:string[][])  [unwired: 2 in, 2 out]
        n216 = local read "Command Params"() -> (w347:string[][])
        n217 = Index Array(array=w352, index (row)=w349, index (col)=0) -> (element=w350:string)
        n218 = call <vilib>:"Invoke Commands.vi"("Command Params"=w347, "Function Name"=w350) -> ("Params"=w346:u8, "Started"=w341:bool)  [unwired: 7 in, 1 out]
        n219 = Array Subset(array=w347, length (row)=w346) -> (w345:string[][])  [unwired: 3 in]
        n220 = Select(t="Executing" ("Cmd Status"), s=w341, f="" ("Cmd Status")) -> (s? t:f=w342:string)
        n221 = local write "Cmd Status"(w342) -> ()
      }
      event "CheckList": Double Click {
        # "Shift clears all"
        # "Update symbols on the listbox"
        n222 = event-data() -> ("PlatMods.Shift"=w355:bool, "Row"=w357:i32)  [unwired: 1 in]
        n223 = case shown="True" w355 {
          tunnel: w357 -> [w361 _]
          tunnel: 1 -> [w360 _]
          frame False {
            n224 = property on="CheckList" class="LstBox (strict)"() -> ("Item Symbols"=w359:i32[])  [unwired: 2 in, 2 out]
            n225 = Replace Array Subset(array=w359, new element=w360, index=w361) -> (w358:i32[])
            n226 = property on="CheckList" class="LstBox (strict)"("Item Symbols"=w358) -> ()  [unwired: 2 in, 2 out]
          }
          frame True {
            w362 = 0 ("Top Row")
            n227 = property on="CheckList" class="LstBox (strict)"() -> ("Number of Rows"=w364:u32)  [unwired: 2 in, 2 out]
            n228 = Initialize Array(0, w364) -> (w363:i32[])
            n229 = property on="CheckList" class="LstBox (strict)"("Top Row"=w362, "Value"=w362, "Item Symbols"=w363) -> ()  [unwired: 2 in, 2 out]
          }
        }
      }
      event "CheckList": Key Down {
        # "Update symbols on the listbox\nLeft and right keys check and uncheck"
        n230 = event-data() -> ("VKey"=w369:T22)  [unwired: 1 in]
        n231 = case shown="\"Left\", \"Right\"" w369 {
          selector: w369 -> [w374 _]
          tunnel: eventvkey."Left" ("VKey") -> [w372 _]
          frame "Left", "Right" {
            n232 = Equal?(x=w372, y=w374) -> (x = y?=w373:bool)
            n233 = Select(t=0, s=w373, f=1) -> (s? t:f=w375:i32)
            n234 = property on="CheckList" class="LstBox (strict)"() -> ("Item Symbols"=w378:i32[])  [unwired: 2 in, 2 out]
            n235 = Replace Array Subset(array=w378, new element=w375, index="CheckList") -> (w377:i32[])
            n236 = property on="CheckList" class="LstBox (strict)"("Item Symbols"=w377) -> ()  [unwired: 2 in, 2 out]
          }
          frame Default {
          }
        }
      }
      event "DB Camera Config": Value Change {
        # "Show or hide the cluster of controls, store in ini file"
        n237 = event-data() -> ("NewVal"=w383:bool)  [unwired: 1 in]
        n238 = case shown="False" w383 {
          tunnel: w382 -> [w392 _]
          tunnel: [w385 w403] -> w381
          tunnel: w380 -> [w384 w403]
          frame False {
            w399 = "Camera"
            w402 = FALSE ("Visible")
            n239 = local read "Camera Settings"() -> (w391:T2)
            n240 = Index Array(array=w392) -> (element=w395:cluster{string[]})  [unwired: 1 in]
            n241 = Unbundle(w391) -> ("Frame Rate"=w390:i32, "Compression"=w389:i32, "Size"=w393:u16)
            n242 = Unbundle(w395) -> (w394:string[])
            n243 = Index Array(array=w394, index=w393) -> (element=w388:string)
            n244 = call-poly <vilib>:"Write Key.vi"("section"=w399, "value"=w388, "key"="Size", "refnum"=w384) -> ("refnum out"=w401:T20)  [unwired: 2 in, 5 out]
            n245 = call-poly <vilib>:"Write Key.vi"("section"=w399, "value"=w390, "key"="FrameRate", "refnum"=w401) -> ("refnum out"=w400:T20)  [unwired: 1 in, 6 out]
            n246 = property on="Camera Settings" class="Clust (strict)"("Visible"=w402) -> ()  [unwired: 2 in, 2 out]
            n247 = local write "DB Camera Config"(w402) -> ()
            n248 = call-poly <vilib>:"Write Key.vi"("section"=w399, "value"=w389, "key"="Compression", "refnum"=w400) -> ("refnum out"=w386:T20)  [unwired: 1 in, 6 out]
            n249 = call <vilib>:"Close Config Data.vi"("refnum"=w386) -> ("file path"=w387:path)  [unwired: 2 in, 8 out]
            n250 = call <vilib>:"Open Config Data.vi"("configuration file path"=w387) -> ("refnum"=w385:T20)  [unwired: 8 in, 2 out]
          }
          frame True {
            n251 = property on="Camera Settings" class="Clust (strict)"("Visible"=TRUE) -> ()  [unwired: 2 in, 2 out]
          }
        }
      }
      event "Camera Settings": Value Change {
        # "Update summary string when any elements of DB camera change"
        n252 = event-data() -> ("NewVal"=w417:T2)  [unwired: 1 in]
        n253 = Index Array(array=w413) -> (element=w412:cluster{string[]})  [unwired: 1 in]
        n254 = Unbundle(w417) -> ("Frame Rate"=w408:i32, "Compression"=w407:i32, "Size"=w410:u16)
        n255 = Unbundle(w412) -> (w411:string[])
        n256 = Index Array(array=w411, index=w410) -> (element=w409:string)
        n257 = Format Into String(format string="%s   %dfps   %d%%", w409, w408, w407) -> (resulting string=w414:string)  [unwired: 2 in, 1 out]
        n258 = Build Array(w414) -> (w415:string[])
        n259 = property on="DB Camera Config" class="Bool (strict)"("Strings [4]"=w415) -> ()  [unwired: 2 in, 2 out]
      }
      event "Motor.Enable": Value Change {
        # "When the test mode otor enable helper is set, update that\ntree row item's value"
        n260 = event-data() -> ("NewVal"=w424:bool)  [unwired: 1 in]
        n261 = Unbundle("Motor") -> ("Value"=w423:dbl)  [unwired: 1 out]
        n262 = Select(t=w423, s=w424, f=0.0) -> (s? t:f=w421:dbl)
        n263 = call <vilib>:"NT Write Number.vi"("Numeric"=w421, "Name"=w420) -> ()  [unwired: 9 in, 1 out]
      }
      event "Test Slider": Value Change {
        # "When the test mode slider helper is set, update that\ntree row item's value"
        n264 = event-data() -> ("NewVal"=w428:dbl)  [unwired: 1 in]
        n265 = call <vilib>:"NT Write Number.vi"("Numeric"=w428, "Name"=w429) -> ()  [unwired: 9 in, 1 out]
      }
      event "On/Off": Value Change {
        # "When the test mode on/off helper value is set, update that\ntree row item's value"
        n266 = event-data() -> ("NewVal"=w434:bool)  [unwired: 1 in]
        n267 = Boolean To (0,1)(Boolean=w434) -> (0, 1=w433:i16)
        n268 = call <vilib>:"NT Write Number.vi"("Numeric"=w433, "Name"=w432) -> ()  [unwired: 9 in, 1 out]
      }
      event "Rev/Fwd": Value Change {
        # "When the test mode helper value for relays is set, update that\ntree row item's value"
        n269 = event-data() -> ("NewVal.Forward"=w443:bool, "NewVal.Reverse"=w442:bool)  [unwired: 1 in]
        n270 = Boolean To (0,1)(Boolean=w443) -> (0, 1=w439:i16)
        n271 = Boolean To (0,1)(Boolean=w442) -> (0, 1=w441:i16)
        n272 = Negate(x=w441) -> (-x=w440:i16)
        n273 = Add(x=w439, y=w440) -> (x+y=w438:i16)
        n274 = call <vilib>:"NT Write Number.vi"("Numeric"=w438, "Name"=w437) -> ()  [unwired: 9 in, 1 out]
      }
      event "Test Ring": Value Change {
        # "When a test mode helper value is selected from the ring,\nset the tree item's variable to the string value"
        n275 = event-data() -> ("NewVal"=w448:u16)  [unwired: 1 in]
        n276 = property on="Test Ring" class="Ring (strict)"() -> ("Strings []"=w449:string[])  [unwired: 2 in, 2 out]
        n277 = Index Array(array=w449, index=w448) -> (element=w447:string)
        n278 = call <vilib>:"NT Write String.vi"("String"=w447, "Name"=w446) -> ()  [unwired: 9 in, 1 out]
      }
      event "Rec Mode": Value Change {
        # "Update globals for recording mode and path to read log from.\nClear when logging and let NetworkTables set path for vision to\nuse."
        n279 = event-data() -> ("NewVal"=w461:enum32{"Stop", "Record", "Playback"})  [unwired: 1 in]
        n280 = global write "WPI_DashboardLogging Global.vi" "Logging Filename"(path "") -> ()
        n281 = global write "WPI_DashboardLogging Global.vi" "Recording"(w461) -> ()
        n282 = case shown="\"Playback\"" w461 {
          tunnel: w460 -> [_ w463 w472]
          tunnel: [_ _ w471] -> w457
          tunnel: [_ _ w470] -> _
          tunnel: w455 -> [_ _ w468]
          tunnel: cluster{i32, i32} {-250, 170} -> [_ _ w467]
          tunnel: [_ _ T23 {"Image Size"=TRUE, "Image Type"=TRUE, "Pixel Value"=TRUE, "ROI Information"=TRUE, "Zoom Factor"=FALSE} ("Image Information Shown:All Elements")] -> w453
          tunnel: [_ _ TRUE ("Zoom Factor")] -> w452
          tunnel: w451 -> [_ _ w464]
          frame Default {
          }
          frame "Stop", "Record" {
            # "Place Window too"
            n283 = invoke class="VI" method="FP.Close"(reference=w463) -> (reference out=w462:refnum<vi>)  [unwired: 2 in, 2 out]
            n284 = invoke class="VI" method="Abort VI"(reference=w462) -> ()  [unwired: 2 in, 3 out]
          }
          frame "Playback" {
            n285 = call "Open Playback Panel.vi"("Offset"=w467, "DB VI Ref"=w468, "Playback in"=w472) -> ("Playback out"=w469:refnum<vi>)  [unwired: 8 in]
            n286 = register-events(w469, w464) -> (reference out=w471:refnum<event-registration>, error out=w470:errorcluster)  [unwired: 2 in]
          }
        }
        n287 = property on="Camera Image" class="ImageControl"("Image Information Shown"=w453, "Image Information Visible"=w452) -> ()  [unwired: 2 in, 2 out]
        n288 = call <vilib>:"WPI_DashboardNT Log FieldName Cache.vi"("Operation"=enum16{"Lookup/Add", "Index", "Clear"}."Clear") -> ()  [unwired: 8 in, 3 out]
      }
      event Panel Close {
        w474 = enum32{"Stop", "Record", "Playback"}."Stop" ("Rec Mode")
        # "Playback window has been closed, abort"
        n289 = event-data() -> ()  [unwired: 1 in, 4 out]
        n290 = local write "Rec Mode"(w474) -> ()
        n291 = global write "WPI_DashboardLogging Global.vi" "Recording"(w474) -> ()
      }
      event Panel Close {
        # "Abort playback window and ourself"
        n292 = event-data() -> ()  [unwired: 1 in, 4 out]
        n293 = invoke class="VI" method="FP.Close"(reference=w480) -> (reference out=w479:refnum<vi>)  [unwired: 2 in, 2 out]
        n294 = invoke class="VI" method="Abort VI"(reference=w479) -> (error out=w478:errorcluster)  [unwired: 2 in, 2 out]
        n295 = invoke class="VI" method="Abort VI"(error in=w478) -> ()  [unwired: 2 in, 3 out]
      }
      event User Event {
        n296 = event-data() -> ("IDs"=w488:cluster{"RPC field ID":u16, "Unique ID":u16}, "String"=w487:string)  [unwired: 1 in]
        n297 = Bundle("IDs"=w488, "String"=w487) -> (w486:T9)  [unwired: 1 in]
        n298 = call <vilib>:"Retrieve RPC Response.vi"("RPC Response"=w486) -> ("Output"=w483:string[][])  [unwired: 10 in]
        n299 = Build Array (concatenate)(w481, w483) -> (w482:string[][])
        n300 = local write "Command Params"(w482) -> ()
        n301 = local write "Cmd Status"("" ("Cmd Status")) -> ()
      }
      event "Vision": Value Change {
        # "Enable/Disable Compression slider.\nHW USB is hard-coded into the camera"
        n302 = event-data() -> ("NewVal"=w495:u16)  [unwired: 1 in]
        n303 = Equal?(x=w495, y=u32 2 ("milliseconds to wait")) -> (x = y?=w493:bool)
        n304 = Select(t=T24."Disabled and Grayed Out" ("Disabled"), s=w493, f=T24."Enabled" ("Disabled")) -> (s? t:f=w490:T24)
        n305 = property on="Compression" class="Slide (strict)"("DisabledEnum"=w490) -> ()  [unwired: 2 in, 2 out]
      }
    }
  }
  n306 = while {
    tunnel: w47 -> [w498]
    i -> [w501]
    stop <- FALSE stop-if-true
    n307 = Wait (ms)(milliseconds to wait=u32 100) -> ()  [unwired: 1 out]
    n308 = case shown="\"Playback\"" "Rec Mode" {
      tunnel: w501 -> [_ _ w516]
      tunnel: [u32 2829099 ("Base Color") u32 11141120 ("Target Color") w505] -> w497
      frame "Stop", Default {
        # "Reset the color, extra updates don't cost much"
      }
      frame "Record" {
      }
      frame "Playback" {
        # "Playback"
        n309 = Quotient & Remainder(x=w516, y=u32 50 ("milliseconds to wait")) -> (x-y*floor(x/y)=w512:u32)  [unwired: 1 out]
        n310 = Divide(x=w512, y=u32 50 ("milliseconds to wait")) -> (x/y=w509:dbl)
        n311 = Multiply(x=6.283185307179586, y=w509) -> (x*y=w514:dbl)
        n312 = Sine(x=w514) -> (sin(x)=w513:dbl)
        n313 = Absolute Value(x=w513) -> (abs(x)=w506:dbl)
        n314 = call "Interpolate RGB Color.vi"("Proportion"=w506, "Target Color"=u32 30976, "Base Color"=u32 2829099) -> ("Result Color"=w505:u32)  [unwired: 8 in]
      }
    }
    n315 = property class="Pane"(reference=w498, "PaneColor"=w497) -> ()  [unwired: 1 in, 2 out]
  }
  n316 = local write "Dashboard Tab"(T1."Drive" ("Dashboard Tab")) -> ()
  n317 = property on="On/Off" class="Bool (strict)"("Visible"=w15) -> ()  [unwired: 2 in, 2 out]
  n318 = property on="Motor" class="Clust (strict)"("Visible"=w15) -> ()  [unwired: 2 in, 2 out]
  n319 = property on="Progress" class="Clust (strict)"("Visible"=w15) -> ()  [unwired: 2 in, 2 out]
  n320 = property on="Test Ring" class="Ring (strict)"("Visible"=w15) -> ()  [unwired: 2 in, 2 out]
  n321 = property on="Rev/Fwd" class="Clust (strict)"("Visible"=w15) -> ()  [unwired: 2 in, 2 out]
  n322 = property on="Camera Settings" class="Clust (strict)"("Visible"=w15) -> ()  [unwired: 2 in, 2 out]
  n323 = while {
    tunnel: u16 1741 ("timeout ms (25000)") -> [w518]
    stop <- FALSE stop-if-true
    n324 = TCP Create Listener(10:w518) -> (0:w517:errorcluster, 3:w519:refnum<k5>)  [unwired: 4 in, 1 out]
    n325 = case shown="No Error" w517 {
      selector: w517 -> [w521 _]
      tunnel: w519 -> [w522 _]
      frame No Error {
        n326 = while {
          tunnel: w522 -> [w525]
          tunnel: w521 -> [w524]
          stop <- FALSE stop-if-true
          n327 = TCP Wait On Listener(8:w524, 11:w525) -> (0:w526:errorcluster, 4:w527:refnum<k5>)  [unwired: 2 in, 3 out]
          n328 = local write "TCP"(w527) -> ()
          n329 = case shown="No Error" w526 {
            frame No Error {
            }
            frame Error {
              n330 = Wait (ms)(milliseconds to wait=u32 1000) -> ()  [unwired: 1 out]
            }
          }
        }
      }
      frame Error {
        n331 = Wait (ms)(milliseconds to wait=u32 1000) -> ()  [unwired: 1 out]
      }
    }
  }
  n332 = local write "DB Camera Config"(w15) -> ()
  n333 = local write "Command Params"(string[][] [] ("Command Params")) -> ()
  n334 = global write "WPI_DashboardLogging Global.vi" "Recording"(w41) -> ()
  n335 = local write "Command Selection"(u16 0 ("milliseconds to wait")) -> ()
  n336 = local write "Rec Mode"(w41) -> ()
